vi "Lakeshore_monitor.vi"(7 "error? 2":errorcluster, 10 "VISA Resource (TPX)":refnum<visa-resource-name>="LakeShore336") -> (0 "error?":errorcluster, 1 "Outputs":T1 {"Heater 1 Output 2" format="%_3g"; "Heater 2 Output 1" format="%_3g"}, 2 "Inputs":T2 {"A:  Sample Stage" format="%_6g"; "B:  Rad Shield" format="%_6g"}, 3 "VISA resource name":refnum<visa-resource-name>)   [LabVIEW 2012]
uses:
  Instrument Libraries/Lake Shore 336/Lake Shore 336.lvlib
  Instrument Libraries/Lake Shore 336/Public/Data/Sensor Data (Single Reading).vi
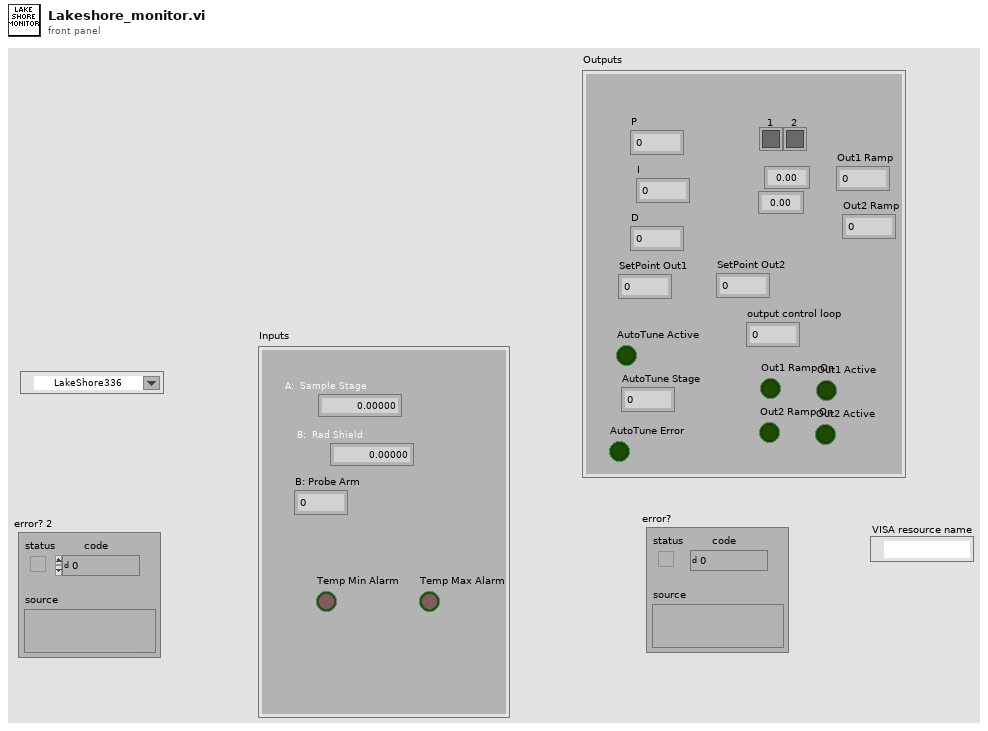
[diagram p1: front panel]
types:
  T1 = cluster{"P":dbl, "I":dbl, "D":dbl, "SetPoint Out1":dbl, "SetPoint Out2":dbl, "1":bool, "2":bool, "output control loop":dbl, "AutoTune Error":bool, "AutoTune Active":bool, "AutoTune Stage":dbl, "Out1 Active":bool, "Out1 Ramp On":bool, "Out2 Active":bool, "Out2 Ramp On":bool, "Heater 2 Output 1":dbl, "Heater 1 Output 2":dbl, "Out1 Ramp":dbl, "Out2 Ramp":dbl}
  T2 = cluster{"A:  Sample Stage":dbl, "B:  Rad Shield":dbl, "B: Probe Arm":dbl, "Temp Max Alarm":bool, "Temp Min Alarm":bool}
  T3 = cluster{"Sensor Data":dbl, "Sensor Data":dbl, "Sensor Data":dbl, "High Alarm Active?":bool, "Low Alarm Active?":bool}
  T4 = cluster{"Gain (P)":dbl, "Reset (I)":dbl, "Rate (D)":dbl, "Setpoint":dbl, "Setpoint":dbl, bool, bool, "Output's Control Loop":u16, "Tuning Error?":bool, "Tuning Active?":bool, "Stage Status":u16, "Ramping Active?":bool, "Ramping On?":bool, "Ramping Active?":bool, "Ramping On?":bool, "Output Value":dbl, "Output Value":dbl, "Ramp Rate":dbl, "Ramp Rate":dbl}
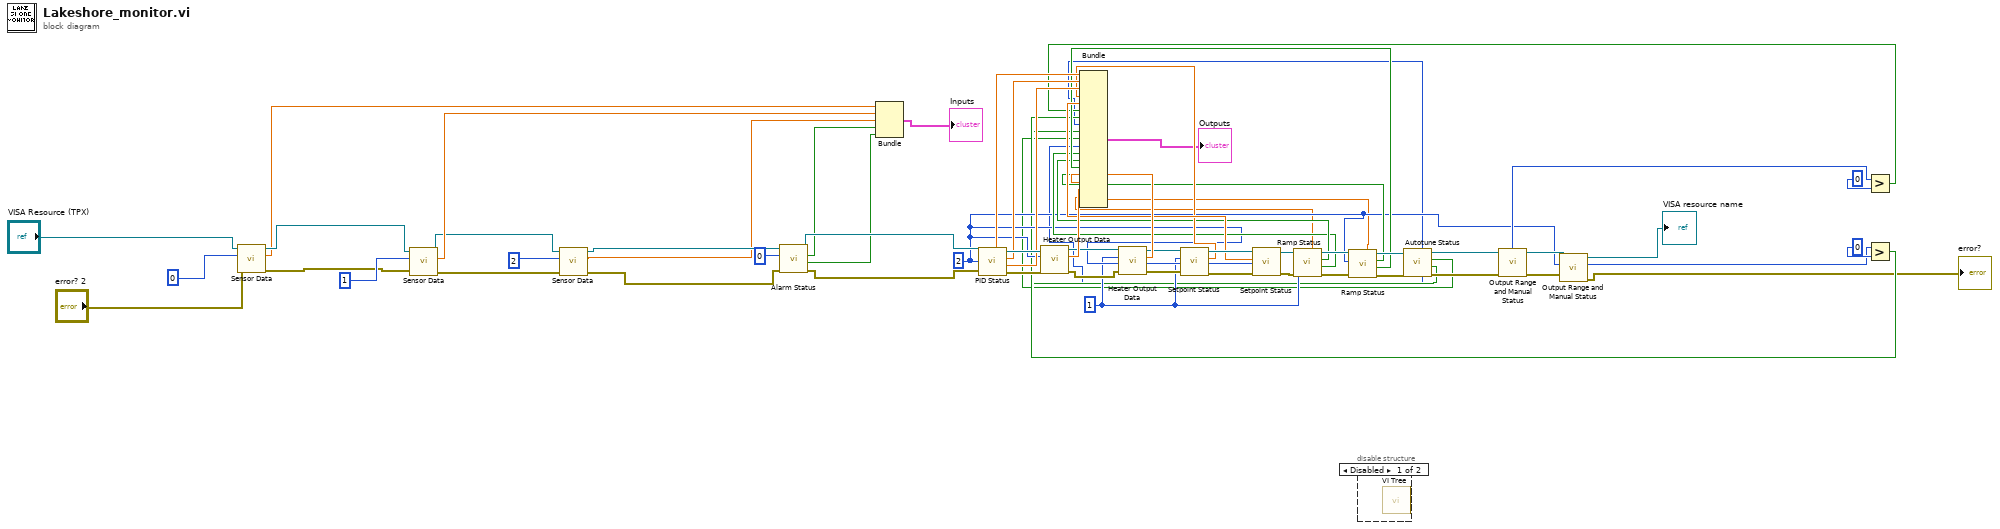
[diagram p0: block diagram]
diagram:
  w23 = 1
  w24 = 2
  n1 = call-poly "Sensor Data.vi"("error in (no error)"="error? 2", "Input (0:A)"=0, "VISA resource name"="VISA Resource (TPX)") -> ("error out"=w59:errorcluster, "Sensor Data"=w53:dbl, "VISA resource name out"=w60:refnum<visa-resource-name>)  [unwired: 6 in]
  n2 = call-poly "Sensor Data.vi"("error in (no error)"=w59, "Input (0:A)"=1, "VISA resource name"=w60) -> ("error out"=w2:errorcluster, "Sensor Data"=w52:dbl, "VISA resource name out"=w6:refnum<visa-resource-name>)  [unwired: 6 in]
  n3 = call-poly "Sensor Data.vi"("error in (no error)"=w2, "Input (0:A)"=2, "VISA resource name"=w6) -> ("error out"=w3:errorcluster, "Sensor Data"=w4:dbl, "VISA resource name out"=w5:refnum<visa-resource-name>)  [unwired: 6 in]
  n4 = call "Alarm Status.vi"("error in (no error)"=w3, "Input (0:A)"=0, "VISA resource name"=w5) -> ("error out"=w56:errorcluster, "Low Alarm Active?"=w50:bool, "High Alarm Active?"=w51:bool, "VISA resource name out"=w57:refnum<visa-resource-name>)  [unwired: 5 in]
  n5 = Bundle("Sensor Data"=w53, "Sensor Data"=w52, "Sensor Data"=w4, "High Alarm Active?"=w51, "Low Alarm Active?"=w50) -> (→"Inputs":T3)  [unwired: 1 in]
  n6 = call "PID Status.vi"("error in (no error)"=w56, "Output's Control Loop (1:1)"=w24, "VISA resource name"=w57) -> ("error out"=w54:errorcluster, "Rate (D)"=w46:dbl, "Reset (I)"=w47:dbl, "VISA resource name out"=w55:refnum<visa-resource-name>, "Gain (P)"=w48:dbl)  [unwired: 4 in]
  n7 = call "Heater Output Data.vi"("error in (no error)"=w54, "Heater Output (1:1)"=w24, "VISA resource name"=w55) -> ("error out"=w43:errorcluster, "Output Value"=w45:dbl, "VISA resource name out"=w44:refnum<visa-resource-name>)  [unwired: 6 in]
  n8 = call "Heater Output Data.vi"("error in (no error)"=w43, "Heater Output (1:1)"=w23, "VISA resource name"=w44) -> ("error out"=w38:errorcluster, "Output Value"=w42:dbl, "VISA resource name out"=w39:refnum<visa-resource-name>)  [unwired: 6 in]
  n9 = call "Setpoint Status.vi"("error in (no error)"=w38, "Output (1:1)"=w23, "VISA resource name"=w39) -> ("error out"=w41:errorcluster, "Setpoint"=w36:dbl, "VISA resource name out"=w40:refnum<visa-resource-name>)  [unwired: 6 in]
  n10 = call "Setpoint Status.vi"("error in (no error)"=w41, "Output (1:1)"=w24, "VISA resource name"=w40) -> ("error out"=w66:errorcluster, "Setpoint"=w37:dbl, "VISA resource name out"=w65:refnum<visa-resource-name>)  [unwired: 6 in]
  n11 = call "Ramp Status.vi"("error in (no error)"=w66, "Output's Control Loop (1:1)"=w23, "VISA resource name"=w65) -> ("error out"=w34:errorcluster, "Ramping Active?"=w28:bool, "Ramping On?"=w29:bool, "VISA resource name out"=w35:refnum<visa-resource-name>, "Ramp Rate"=w19:dbl)  [unwired: 4 in]
  n12 = call "Ramp Status.vi"("error in (no error)"=w34, "Output's Control Loop (1:1)"=w24, "VISA resource name"=w35) -> ("error out"=w32:errorcluster, "Ramping Active?"=w30:bool, "Ramping On?"=w31:bool, "VISA resource name out"=w33:refnum<visa-resource-name>, "Ramp Rate"=w18:dbl)  [unwired: 4 in]
  n13 = disable-structure shown="Disabled" {
    frame Disabled {
      n14 = call "VI Tree.vi"() -> ()  [unwired: 12 in]
    }
    frame Enabled {
    }
  }
  n15 = call "Autotune Status.vi"("error in (no error)"=w32, "VISA resource name"=w33) -> ("error out"=w15:errorcluster, "Tuning Error?"=w13:bool, "Tuning Active?"=w12:bool, "VISA resource name out"=w16:refnum<visa-resource-name>, "Stage Status"=w11:u16, "Output's Control Loop"=w14:u16)  [unwired: 4 in]
  n16 = call "Output Range and Manual Status.vi"("error in (no error)"=w15, "VISA resource name"=w16) -> ("error out"=w25:errorcluster, "Range (0:Off)"=w27:u16, "VISA resource name out"=w26:refnum<visa-resource-name>)  [unwired: 6 in, 1 out]
  n17 = call "Output Range and Manual Status.vi"("error in (no error)"=w25, "Output (1:1)"=w24, "VISA resource name"=w26) -> ("error out"=→"error?":errorcluster, "Range (0:Off)"=w22:u16, "VISA resource name out"=→"VISA resource name":refnum<visa-resource-name>)  [unwired: 5 in, 1 out]
  n18 = Greater?(x=w27, y=0) -> (0:w21:bool)
  n19 = Greater?(x=w22, y=0) -> (0:w20:bool)
  n20 = Bundle("Gain (P)"=w48, "Reset (I)"=w47, "Rate (D)"=w46, "Setpoint"=w36, "Setpoint"=w37, w21, w20, "Output's Control Loop"=w14, "Tuning Error?"=w13, "Tuning Active?"=w12, "Stage Status"=w11, "Ramping Active?"=w28, "Ramping On?"=w29, "Ramping Active?"=w30, "Ramping On?"=w31, "Output Value"=w42, "Output Value"=w45, "Ramp Rate"=w19, "Ramp Rate"=w18) -> (→"Outputs":T4)  [unwired: 1 in]
